vi "DSA All IO Synch Trig Export.vi"() -> ()   [LabVIEW 2018]
doc: "This example demonstrates how to acquire a continuous amount of data (Waveform) using the DAQ device's internal clock. It also shows how to synchronize two devices for different device families (E Series, S Series, M Series, X Series, DSA, and SC Express), to simultaneously acquire the data.\n\nFor instructions on how to connect your signals to the DAQ device, refer to your device documentation."
uses:
  <vilib>/Utility/error.llb/DialogType.ctl
  <vilib>/DAQmx/write.llb/DAQmx Write (Analog 1D Wfm NChan NSamp).vi
  <vilib>/DAQmx/read.llb/DAQmx Read (Analog 1D Wfm NChan NSamp).vi
  <vilib>/DAQmx/create/channels.llb/DAQmx Create Channel (AO-Voltage-Basic).vi
  <vilib>/DAQmx/configure/timing.llb/DAQmx Timing (Sample Clock).vi
  <vilib>/DAQmx/create/channels.llb/DAQmx Create Channel (AI-Voltage-Basic).vi
  <vilib>/DAQmx/configure/trigger.llb/DAQmx Start Trigger (Digital Edge).vi
  <vilib>/DAQmx/miscellaneous.llb/DAQmx Fill In Error Info.vi
  <vilib>/measure/matone.llb/Extract Single Tone Information N Chan.vi
  <resource>/objmgr/daqmx.rc
  <vilib>/measure/NI_MABase.lvlib
  <vilib>/measure/NI_MAPro.lvlib
panel:
  in  "error in":errorcluster
  in  "/PXIe-6341/PXI_Trig0":tag="/PXIe-6341/PXI_Trig0"
  in  "/PXIe-6341/PFI0":tag="/PXIe-6341/PFI0"
  in  "/PXI-4461/PXI_Trig0":tag="/PXI-4461/PXI_Trig0"
  in  "/PXI-4461/ai/StartTrigger":tag="/PXI-4461/ai/StartTrigger"
  out "Waveform Graph 2":dbl[](graph)
  in  "PXI-4461B/ao0:1":tag="PXI-4461B/ao0:1"
  in  "Output Array":T1(array[cluster])=[{"Waveform Type"=0, "Amplitude"=0.01, "Frequency"=10.0}, {"Waveform Type"=0, "Amplitude"=0.01, "Frequency"=10.0}] {"Frequency" format="%0.2p"; "Amplitude" format="%0.2p"; "Waveform Type" items=["Sine Wave", "Triangle Wave", "Square Wave", "Sawtooth Wave"]}
  in  "Number of Samples":i32=48000
  in  "PXI-4461/ao0:1":tag="PXI-4461/ao0:1"
  in  "Stop":bool
  out "Waveform Graph":waveform(dbl)[](graph)
  in  "Samples per Loop":i32=4800
  in  "Sample Rate":dbl=48000.0
  in  "PXI-4461/ai0:1, PXI-4461B/ai0:1":tag="PXI-4461/ai0:1, PXI-4461B/ai0:1"
  # "*Note:  This example is intended to show low level synchronization of various devices.\nDSA, S Series, X Series, and SC Express devices support including channels from multiple devices in a single task.\nDAQmx automatically synchronizes the devices in such a task.  See the DAQmx Help>>\nDevice Considerations>>Multi Device Tasks section for further details."
  # "Channel Settings"
  # "Acquired Data"
  # "Timing Settings"
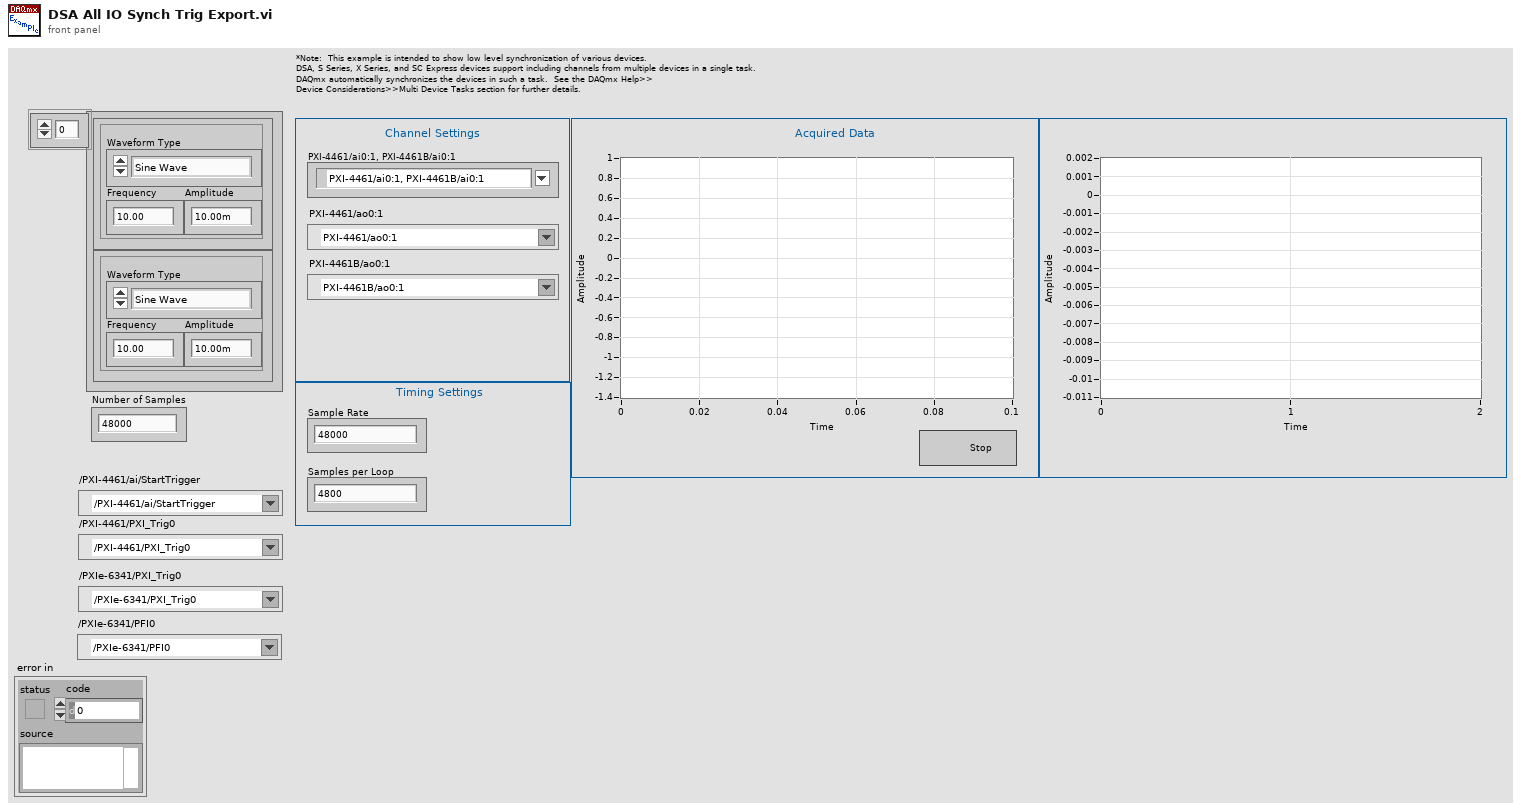
[diagram p1: front panel]
types:
  T1 = cluster{"Waveform Type":u16, "Amplitude":dbl, "Frequency":dbl}[]
  T2 = typedef "DialogType.ctl" = u16
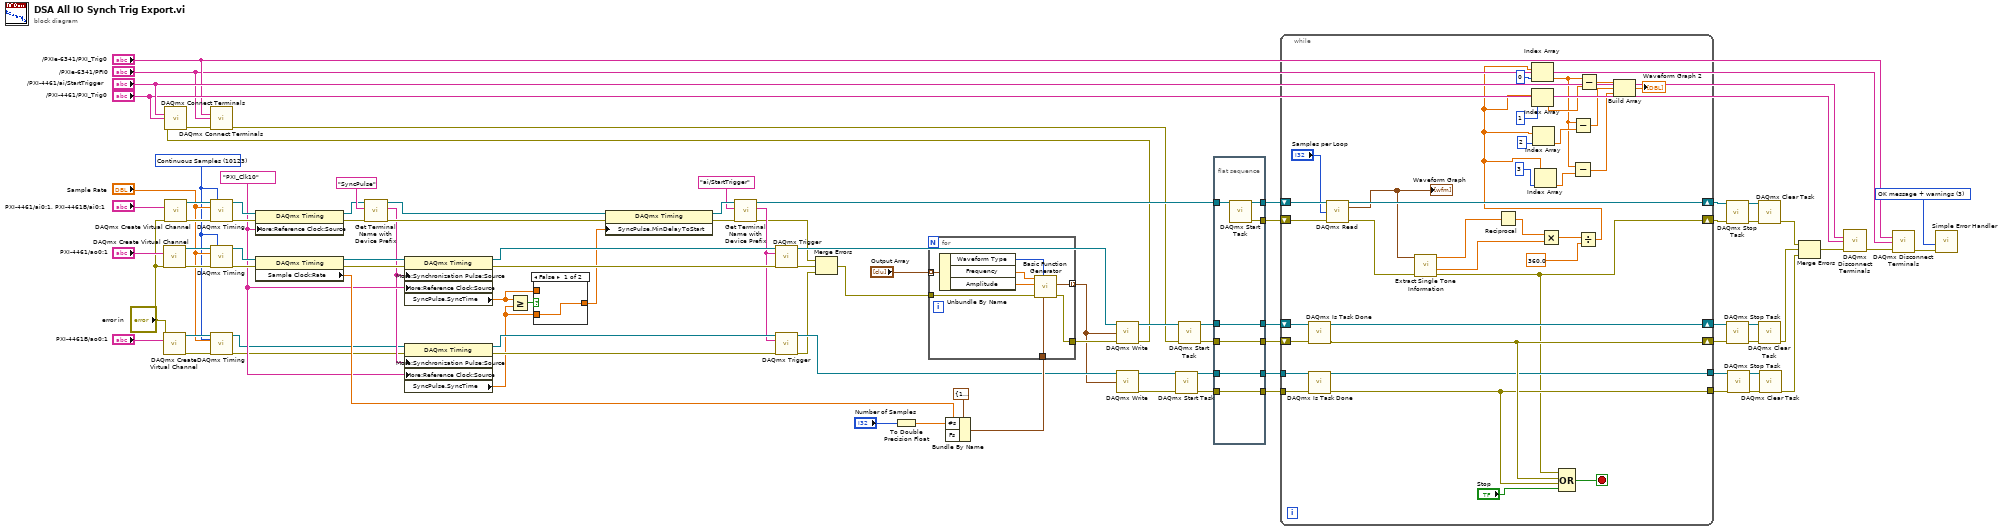
[diagram p0: block diagram]
diagram:
  w11 = tag "PXI_Clk10" ("RefClk.Src")
  w64 = T2 3 items=["no dialog", "OK message", "continue or stop message", "OK message + warnings", "continue/stop + warnings"] ("type of dialog (OK msg:1)")
  w45 = 10123 items=["Finite Samples"=10178, "Continuous Samples"=10123, "Hardware Timed Single Point"=12522] ("Sample Mode")
  n1 = call-poly <vilib>:"DAQmx Create Virtual Channel.vi"("physical channels"="PXI-4461/ao0:1", "error in"="error in") -> ("task out"=w71:refnum<k21>, "error out"=w72:errorcluster)  [unwired: 12 in]
  n2 = call-poly <vilib>:"DAQmx Create Virtual Channel.vi"("physical channels"="PXI-4461B/ao0:1", "error in"="error in") -> ("task out"=w48:refnum<k21>, "error out"=w47:errorcluster)  [unwired: 12 in]
  n3 = call-poly <vilib>:"DAQmx Create Virtual Channel.vi"("physical channels"="PXI-4461/ai0:1, PXI-4461B/ai0:1", "error in"="error in") -> ("task out"=w76:refnum<k21>, "error out"=w75:errorcluster)  [unwired: 12 in]
  n4 = call-poly <vilib>:"DAQmx Timing.vi"("task/channels in"=w76, "sample mode"=w45, "rate"="Sample Rate", "error in"=w75) -> ("task out"=w73:refnum<k21>, "error out"=w74:errorcluster)  [unwired: 10 in]
  n5 = call-poly <vilib>:"DAQmx Timing.vi"("task/channels in"=w71, "sample mode"=w45, "rate"="Sample Rate", "error in"=w72) -> ("task out"=w63:refnum<k21>, "error out"=w61:errorcluster)  [unwired: 10 in]
  n6 = call-poly <vilib>:"DAQmx Timing.vi"("task/channels in"=w48, "sample mode"=w45, "rate"="Sample Rate", "error in"=w47) -> ("task out"=w9:refnum<k21>, "error out"=w8:errorcluster)  [unwired: 10 in]
  n7 = property class="DAQmx Timing"(reference=w73, error in=w74, "More:Reference Clock:Source"=w11) -> (reference out=w19:refnum<k21>, error out=w18:errorcluster)
  n8 = property class="DAQmx Timing"(reference=w63, error in=w61) -> (reference out=w62:refnum<k21>, error out=w60:errorcluster, "Sample Clock:Rate"=w50:dbl)
  n9 = call "Get Terminal Name with Device Prefix.vi"("error in"=w18, "Local Terminal Name"="SyncPulse", "task/channels in"=w19) -> ("error out"=w16:errorcluster, "Terminal Name with Device Prefix"=w10:tag, "task out"=w17:refnum<k21>)  [unwired: 6 in]
  n10 = property class="DAQmx Timing"(reference=w62, error in=w60, "More:Synchronization Pulse:Source"=w10, "More:Reference Clock:Source"=w11) -> (reference out=w70:refnum<k21>, error out=w69:errorcluster, "SyncPulse.SyncTime"=w14:dbl)
  n11 = property class="DAQmx Timing"(reference=w9, error in=w8, "More:Synchronization Pulse:Source"=w10, "More:Reference Clock:Source"=w11) -> (reference out=w44:refnum<k21>, error out=w43:errorcluster, "SyncPulse.SyncTime"=w12:dbl)
  n12 = Greater Or Equal?(x=w14, y=w12) -> (x >= y?=w15:bool)
  n13 = case shown="False" w15 {
    tunnel: w14 -> [_ w95]
    tunnel: [w94 w95] -> w13
    tunnel: w12 -> [w94 _]
    frame False {
    }
    frame True {
    }
  }
  n14 = property class="DAQmx Timing"(reference=w17, error in=w16, "SyncPulse.MinDelayToStart"=w13) -> (reference out=w68:refnum<k21>, error out=w67:errorcluster)
  n15 = call "Get Terminal Name with Device Prefix.vi"("error in"=w67, "Local Terminal Name"="ai/StartTrigger", "task/channels in"=w68) -> ("error out"=w6:errorcluster, "Terminal Name with Device Prefix"=w29:tag, "task out"=w66:refnum<k21>)  [unwired: 6 in]
  n16 = call-poly <vilib>:"DAQmx Trigger.vi"("task/channels in"=w70, "source"=w29, "error in"=w69) -> ("task out"=w51:refnum<k21>, "error out"=w4:errorcluster)  [unwired: 11 in]
  n17 = call-poly <vilib>:"DAQmx Trigger.vi"("task/channels in"=w44, "source"=w29, "error in"=w43) -> ("task out"=w42:refnum<k21>, "error out"=w5:errorcluster)  [unwired: 11 in]
  n18 = Merge Errors(w6, w4, w5) -> (w3:errorcluster)
  n19 = To Double Precision Float(number="Number of Samples") -> (double precision float=w54:dbl)
  n20 = Bundle By Name(cluster=cluster{"Fs":dbl, "#s":dbl} {"Fs"=1000.0, "#s"=1000.0} ("sampling info"), "#s"=w54, "Fs"=w50) -> (w57:cluster{"Fs":dbl, "#s":dbl})
  n21 = for {
    tunnel: w3 -> [w103]
    tunnel: w57 -> [w102]
    tunnel: [w101] -> w56
    tunnel: "Output Array" -> [w100] mode=indexing
    tunnel: [w96] -> w41 mode=indexing
    n22 = Unbundle By Name(w100) -> ("Waveform Type"=w99:u16, "Frequency"=w98:dbl, "Amplitude"=w97:dbl)
    n23 = call <vilib>:"Basic Function Generator.vi"("sampling info"=w102, "signal type"=w99, "error in (no error)"=w103, "amplitude"=w97, "frequency"=w98) -> ("error out"=w101:errorcluster, "signal out"=w96:waveform(dbl))  [unwired: 4 in, 1 out]
  }
  n24 = call-poly <vilib>:"DAQmx Write.vi"("task/channels in"=w51, "data"=w41, "error in"=w56) -> ("task out"=w52:refnum<k21>, "error out"=w2:errorcluster)  [unwired: 10 in, 1 out]
  n25 = call <vilib>:"DAQmx Connect Terminals.vi"("source terminal"="/PXI-4461/ai/StartTrigger", "destination terminal"="/PXI-4461/PXI_Trig0", "error in"=w2) -> ("error out"=w28:errorcluster)  [unwired: 12 in]
  n26 = call <vilib>:"DAQmx Connect Terminals.vi"("source terminal"="/PXIe-6341/PXI_Trig0", "destination terminal"="/PXIe-6341/PFI0", "error in"=w28) -> ("error out"=w1:errorcluster)  [unwired: 12 in]
  n27 = call-poly <vilib>:"DAQmx Write.vi"("task/channels in"=w42, "data"=w41) -> ("task out"=w40:refnum<k21>, "error out"=w39:errorcluster)  [unwired: 11 in, 1 out]
  n28 = call <vilib>:"DAQmx Start Task.vi"("task/channels in"=w40, "error in"=w39) -> ("task out"=w38:refnum<k21>, "error out"=w37:errorcluster)  [unwired: 12 in]
  n29 = call <vilib>:"DAQmx Start Task.vi"("task/channels in"=w52, "error in"=w1) -> ("task out"=w93:refnum<k21>, "error out"=w92:errorcluster)  [unwired: 12 in]
  n30 = flat-sequence {
    tunnel: w93 -> [w110]
    tunnel: w92 -> [w109]
    tunnel: [w110] -> w89
    tunnel: [w109] -> w88
    tunnel: [w108] -> w90
    tunnel: [w107] -> w91
    tunnel: w66 -> [w106]
    tunnel: w38 -> [w105]
    tunnel: w37 -> [w104]
    tunnel: [w105] -> w36
    tunnel: [w104] -> w35
    frame #0 {
      n31 = call <vilib>:"DAQmx Start Task.vi"("task/channels in"=w106) -> ("task out"=w107:refnum<k21>, "error out"=w108:errorcluster)  [unwired: 13 in]
    }
  }
  n32 = while {
    shift-right: [w129] -> w86
    shift-left: w90 -> [w142]
    shift-right: [w138] -> w82
    shift-left: w88 -> [w139]
    shift-right: [w144] -> w87
    shift-left: w91 -> [w143]
    shift-right: [w137] -> w83
    shift-left: w89 -> [w140]
    tunnel: w36 -> [w136]
    tunnel: w35 -> [w135]
    tunnel: [w133] -> w32
    tunnel: [w132] -> w31
    stop <- w145 stop-if-true
    n33 = call <vilib>:"DAQmx Is Task Done.vi"("task/channels in"=w140, "error in"=w139) -> ("task out"=w137:refnum<k21>, "error out"=w138:errorcluster)  [unwired: 11 in, 1 out]
    n34 = call <vilib>:"DAQmx Is Task Done.vi"("task/channels in"=w136, "error in"=w135) -> ("task out"=w133:refnum<k21>, "error out"=w132:errorcluster)  [unwired: 11 in, 1 out]
    n35 = call-poly <vilib>:"DAQmx Read.vi"("task/channels in"=w143, "number of samples per channel"="Samples per Loop", "error in"=w142) -> ("task out"=w144:refnum<k21>, "data"=w131:waveform(dbl)[], "error out"=w130:errorcluster)  [unwired: 10 in]
    "Waveform Graph" <- w131
    n36 = call-poly <vilib>:"Extract Single Tone Information.vi"("error in (no error)"=w130, "time signals in"=w131) -> ("error out"=w129:errorcluster, "detected phases (deg)"=w116:dbl[], "detected frequencies"=w117:dbl[])  [unwired: 4 in, 3 out]
    n37 = Reciprocal(x=w117) -> (1/x=w118:dbl[])
    n38 = Multiply(x=w118, y=w116) -> (x*y=w115:dbl[])
    n39 = Compound Arithmetic op=OR(w129, w138, w132, "Stop") -> (w145:bool)
    n40 = Divide(x=w115, y=360.0) -> (x/y=w113:dbl[])
    n41 = Index Array(array=w113, index=0) -> (element=w121:dbl)
    n42 = Index Array(array=w113, index=1) -> (element=w126:dbl)
    n43 = Index Array(array=w113, index=2) -> (element=w123:dbl)
    n44 = Index Array(array=w113, index=3) -> (element=w122:dbl)
    n45 = Subtract(x=w121, y=w122) -> (x-y=w119:dbl)
    n46 = Subtract(x=w121, y=w123) -> (x-y=w120:dbl)
    n47 = Subtract(x=w121, y=w126) -> (x-y=w112:dbl)
    n48 = Build Array(w112, w120, w119) -> (→"Waveform Graph 2":dbl[])
  }
  n49 = call <vilib>:"DAQmx Stop Task.vi"("task/channels in"=w87, "error in"=w86) -> ("task out"=w84:refnum<k21>, "error out"=w85:errorcluster)  [unwired: 12 in]
  n50 = call <vilib>:"DAQmx Stop Task.vi"("task/channels in"=w83, "error in"=w82) -> ("task out"=w80:refnum<k21>, "error out"=w81:errorcluster)  [unwired: 12 in]
  n51 = call <vilib>:"DAQmx Stop Task.vi"("task/channels in"=w32, "error in"=w31) -> ("task out"=w34:refnum<k21>, "error out"=w33:errorcluster)  [unwired: 12 in]
  n52 = call <vilib>:"DAQmx Clear Task.vi"("task in"=w84, "error in"=w85) -> ("error out"=w79:errorcluster)  [unwired: 13 in]
  n53 = call <vilib>:"DAQmx Clear Task.vi"("task in"=w80, "error in"=w81) -> ("error out"=w78:errorcluster)  [unwired: 13 in]
  n54 = call <vilib>:"DAQmx Clear Task.vi"("task in"=w34, "error in"=w33) -> ("error out"=w30:errorcluster)  [unwired: 13 in]
  n55 = Merge Errors(w79, w78, w30) -> (w22:errorcluster)
  n56 = call <vilib>:"DAQmx Disconnect Terminals.vi"("source terminal"="/PXI-4461/ai/StartTrigger", "destination terminal"="/PXI-4461/PXI_Trig0", "error in"=w22) -> ("error out"=w27:errorcluster)  [unwired: 12 in]
  n57 = call <vilib>:"DAQmx Disconnect Terminals.vi"("source terminal"="/PXIe-6341/PXI_Trig0", "destination terminal"="/PXIe-6341/PFI0", "error in"=w27) -> ("error out"=w21:errorcluster)  [unwired: 12 in]
  n58 = call <vilib>:"Simple Error Handler.vi"("type of dialog (OK msg:1)"=w64, "error in (no error)"=w21) -> ()  [unwired: 3 in, 5 out]
